vi "Battery_TEST.vi"() -> ()   [LabVIEW 2018]
uses:
  <vilib>/Instr/_visa.llb/VISA Configure Serial Port (Instr).vi
panel:
  out "SOC":u16
  out "Discharge":dbl
  out "Charge":dbl
  out "Batt_Volt":dbl
  in  "COM":refnum<visa-resource-name>="COM6"
  in  "stop":bool
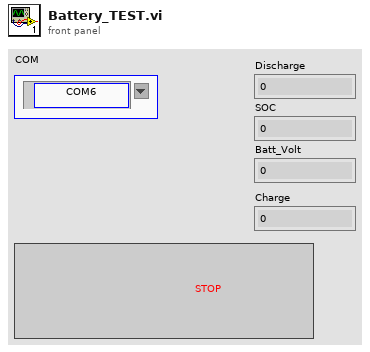
[diagram p1: front panel]
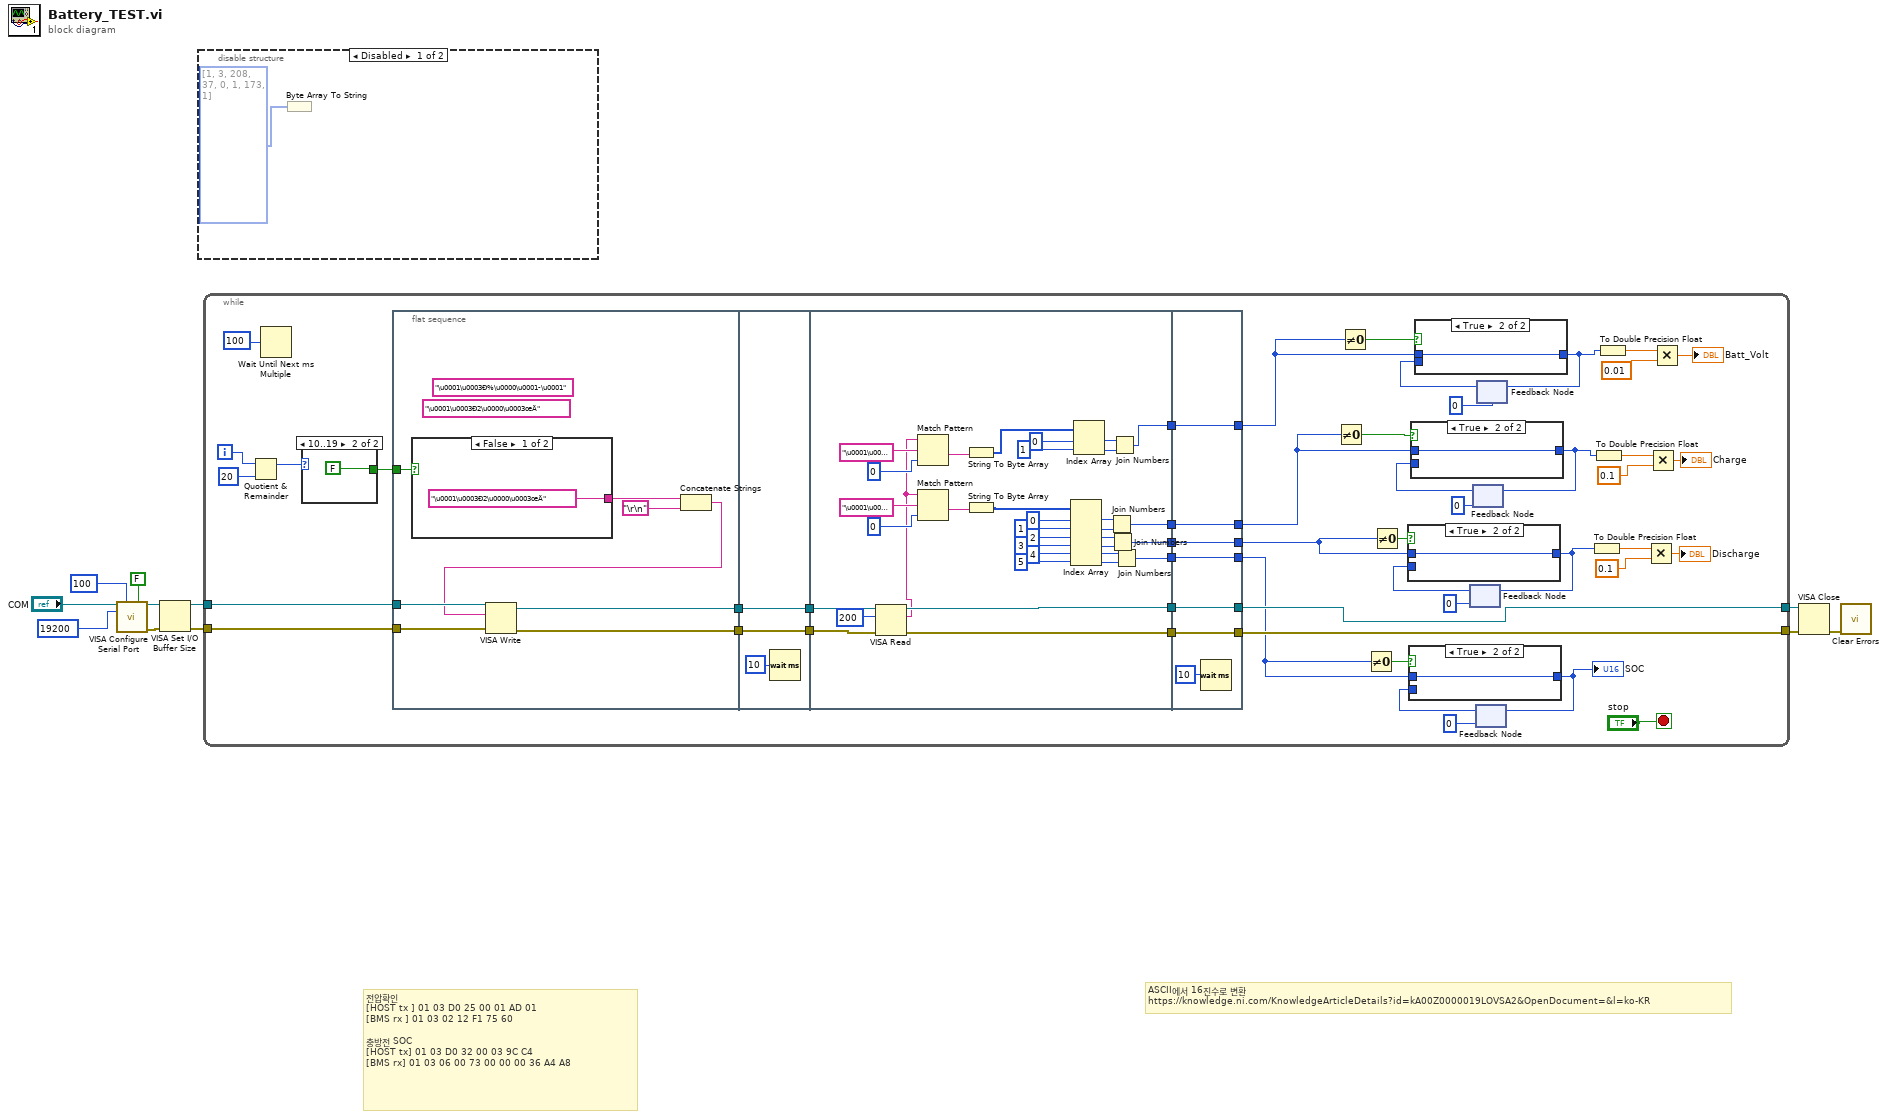
[diagram p0: block diagram]
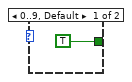
[diagram p7: hidden frame]
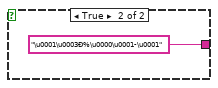
[diagram p8: hidden frame]
diagram:
  # "ASCII에서 16진수로 변환\nhttps://knowledge.ni.com/KnowledgeArticleDetails?id=kA00Z0000019LOVSA2&OpenDocument=&l=ko-KR"
  # "전압확인\n[HOST tx ] 01 03 D0 25 00 01 AD 01\n[BMS rx ] 01 03 02 12 F1 75 60\n\n충방전 SOC\n[HOST tx] 01 03 D0 32 00 03 9C C4\n[BMS rx] 01 03 06 00 73 00 00 00 36 A4 A8"
  n1 = call-poly "VISA Configure Serial Port"("VISA resource name"="COM", "timeout (10sec)"=u32 100, "Enable Termination\nChar (T)"=FALSE ("Enable Termination\nChar (T)"), "baud rate (9600)"=u32 19200 ("baud rate")) -> ("VISA resource name out"=w8:refnum<visa-resource-name>, "error out"=w7:errorcluster)  [unwired: 10 in]
  n2 = VISA Set I/O Buffer Size(VISA resource name=w8, error in (no error)=w7) -> (VISA resource name out=w4:refnum<visa-resource-name>, error out=w3:errorcluster)  [unwired: 2 in]
  n3 = disable-structure shown="Disabled" {
    frame Disabled {
      n4 = Byte Array To String(unsigned byte array=u8[] [1, 3, 208, 37, 0, 1, 173, 1]) -> ()  [unwired: 1 out]
    }
    frame Enabled {
    }
  }
  n5 = while {
    tunnel: w4 -> [w58]
    tunnel: w3 -> [w57]
    tunnel: [w52] -> w6
    tunnel: [w51] -> w5
    i -> [w49]
    stop <- "stop" stop-if-true
    n6 = Quotient & Remainder(x=w49, y=u32 20) -> (x-y*floor(x/y)=w46:u32)  [unwired: 1 out]
    n7 = Wait Until Next ms Multiple(millisecond multiple=u32 100 ("타임아웃(ms) (-1)")) -> ()  [unwired: 1 out]
    n8 = case shown="10..19" w46 {
      tunnel: [TRUE FALSE] -> w47
      frame 0..9, Default {
      }
      frame 10..19 {
      }
    }
    n9 = flat-sequence {
      tunnel: [w79] -> w60
      tunnel: [w78] -> w59
      tunnel: w58 -> [w77]
      tunnel: w57 -> [w76]
      tunnel: w47 -> [w73]
      tunnel: w60 -> [w84]
      tunnel: w59 -> [w83]
      tunnel: [w84] -> w56
      tunnel: [w83] -> w55
      tunnel: w56 -> [w118]
      tunnel: w55 -> [w117]
      tunnel: [w116] -> w54
      tunnel: [w115] -> w53
      tunnel: [w88] -> w45
      tunnel: [w87] -> w31
      tunnel: [w86] -> w30
      tunnel: [w85] -> w29
      tunnel: w54 -> [w124]
      tunnel: w53 -> [w123]
      tunnel: [w124] -> w52
      tunnel: [w123] -> w51
      tunnel: w45 -> [w122]
      tunnel: [w122] -> w41
      tunnel: [w121] -> w27
      tunnel: w31 -> [w121]
      tunnel: [w120] -> w26
      tunnel: w30 -> [w120]
      tunnel: [w119] -> w25
      tunnel: w29 -> [w119]
      frame #0 {
        (unwired) "\u0001\u0003Ð2\u0000\u0003œÄ"
        (unwired) "\u0001\u0003Ð%\u0000\u0001­\u0001"
        n10 = case shown="False" w73 {
          tunnel: ["\u0001\u0003Ð2\u0000\u0003œÄ" "\u0001\u0003Ð%\u0000\u0001­\u0001"] -> w74
          frame False {
          }
          frame True {
          }
        }
        n11 = Concatenate Strings(w74, "\r\n") -> (w75:string)
        n12 = VISA Write(VISA resource name=w77, write buffer=w75, error in (no error)=w76) -> (VISA resource name out=w79:refnum<visa-resource-name>, error out=w78:errorcluster)  [unwired: 1 out]
      }
      frame #1 {
        n13 = Wait (ms)(milliseconds to wait=u32 10) -> ()  [unwired: 1 out]
      }
      frame #2 {
        n14 = VISA Read(VISA resource name=w118, byte count=u32 200, error in (no error)=w117) -> (VISA resource name out=w116:refnum<visa-resource-name>, read buffer=w107:string, error out=w115:errorcluster)  [unwired: 1 out]
        n15 = Match Pattern(string=w107, regular expression="\u0001\u0003\u0002", offset (0)=0 ("offset past match")) -> (after substring=w111:string)  [unwired: 3 out]
        n16 = Match Pattern(string=w107, regular expression="\u0001\u0003\u0006", offset (0)=0 ("offset past match")) -> (after substring=w110:string)  [unwired: 3 out]
        n17 = String To Byte Array(string=w111) -> (unsigned byte array=w104:u8[])
        n18 = String To Byte Array(string=w110) -> (unsigned byte array=w97:u8[])
        n19 = Index Array(array=w97, index #1=0, index #2=1, index #3=2, index #4=3, index #5=4, index #6=5) -> (element #1=w101:u8, element #2=w100:u8, element #3=w92:u8, element #4=w91:u8, element #5=w90:u8, element #6=w89:u8)
        n20 = Index Array(array=w104, index #1=0, index #2=1) -> (element #1=w102:u8, element #2=w103:u8)
        n21 = Join Numbers(hi=w101, lo=w100) -> ((hi.lo)=w87:u16)
        n22 = Join Numbers(hi=w92, lo=w91) -> ((hi.lo)=w86:u16)
        n23 = Join Numbers(hi=w102, lo=w103) -> ((hi.lo)=w88:u16)
        n24 = Join Numbers(hi=w90, lo=w89) -> ((hi.lo)=w85:u16)
      }
      frame #3 {
        n25 = Wait (ms)(milliseconds to wait=u32 10) -> ()  [unwired: 1 out]
      }
    }
    n26 = Not Equal To 0?(x=w27) -> (x != 0?=w40:bool)
    n27 = Not Equal To 0?(x=w41) -> (x != 0?=w42:bool)
    n28 = Not Equal To 0?(x=w25) -> (x != 0?=w34:bool)
    n29 = Not Equal To 0?(x=w26) -> (x != 0?=w35:bool)
    n30 = feedback #1(u16 0) -> (w37:u16)
    n31 = case shown="True" w35 {
      tunnel: w26 -> [_ w65]
      tunnel: [w64 w65] -> w13
      tunnel: w37 -> [w64 _]
      frame False {
      }
      frame True {
      }
    }
    n32 = feedback-in #1(w13) -> ()
    n33 = feedback #2(u16 0) -> (w38:u16)
    n34 = case shown="True" w40 {
      tunnel: w27 -> [_ w67]
      tunnel: [w66 w67] -> w17
      tunnel: w38 -> [w66 _]
      frame False {
      }
      frame True {
      }
    }
    n35 = feedback-in #2(w17) -> ()
    n36 = feedback #3(u16 0) -> (w32:u16)
    n37 = case shown="True" w34 {
      tunnel: w25 -> [_ w63]
      tunnel: [w62 w63] -> w28
      tunnel: w32 -> [w62 _]
      frame False {
      }
      frame True {
      }
    }
    "SOC" <- w28
    n38 = feedback-in #3(w28) -> ()
    n39 = feedback #4(u16 0) -> (w44:u16)
    n40 = case shown="True" w42 {
      tunnel: w41 -> [_ w69]
      tunnel: [w68 w69] -> w21
      tunnel: w44 -> [w68 _]
      frame False {
      }
      frame True {
      }
    }
    n41 = feedback-in #4(w21) -> ()
    n42 = To Double Precision Float(number=w13) -> (double precision float=w16:dbl)
    n43 = To Double Precision Float(number=w17) -> (double precision float=w19:dbl)
    n44 = To Double Precision Float(number=w21) -> (double precision float=w24:dbl)
    n45 = Multiply(x=w16, y=0.1) -> (x*y=→"Discharge":dbl)
    n46 = Multiply(x=w19, y=0.1) -> (x*y=→"Charge":dbl)
    n47 = Multiply(x=w24, y=0.01) -> (x*y=→"Batt_Volt":dbl)
  }
  n48 = VISA Close(VISA resource name=w6, error in (no error)=w5) -> (error out=w2:errorcluster)
  n49 = call <vilib>:"Clear Errors.vi"("error in (no error)"=w2) -> ()  [unwired: 5 in, 2 out]
